vi "Get date from parts.vi"(1 "Year":i32=2021, 2 "Month":i32=4, 3 "Date":i32=24) -> (0 "Date Stamp":timestamp)   [LabVIEW 2015]
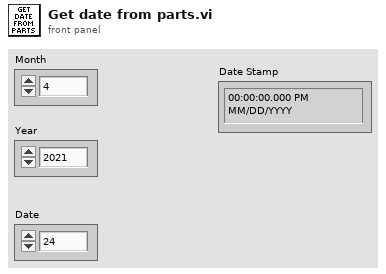
[diagram p1: front panel]
types:
  T1 = typedef "LVDateTimeRec.ctl" = cluster{"fractional second":dbl, "second":i32, "minute":i32, "hour":i32, "day of month":i32, "month":i32, "year":i32, "day of week":i32, "day of year":i32, "DST":i32}
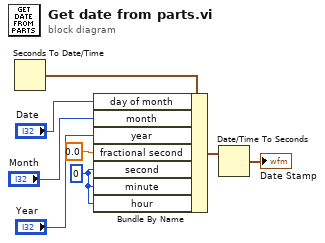
[diagram p0: block diagram]
diagram:
  w6 = 0 ("second")
  n1 = Seconds To Date/Time() -> (date time rec=w8:T1)  [unwired: 2 in]
  n2 = Bundle By Name(cluster=w8, "day of month"="Date", "month"="Month", "year"="Year", "fractional second"=0.0, "second"=w6, "minute"=w6, "hour"=w6) -> (w2:T1)
  n3 = Date/Time To Seconds(2:w2) -> (0:→"Date Stamp":timestamp)  [unwired: 1 in]
